vi "Intensity RMS.vi"(8 "Original Intensity":dbl[][](array[numeric]) format="%0.3f", 9 "Iteration":i32=9, 10 "num rows":i32=256, 11 "field":T1) -> (2 "Best Exponential Fit":dbl[](array[numeric]), 3 "field out":T1)   [LabVIEW 2012, in "LightPipes.lvlib"]
uses:
  LightPipes.lvlib
  <vilib>/Analysis/5stat.llb/RMS (DBL).vi
  <vilib>/Analysis/NI_AALPro.lvlib
  <vilib>/ptbypt/NI_PtbyPt.lvlib
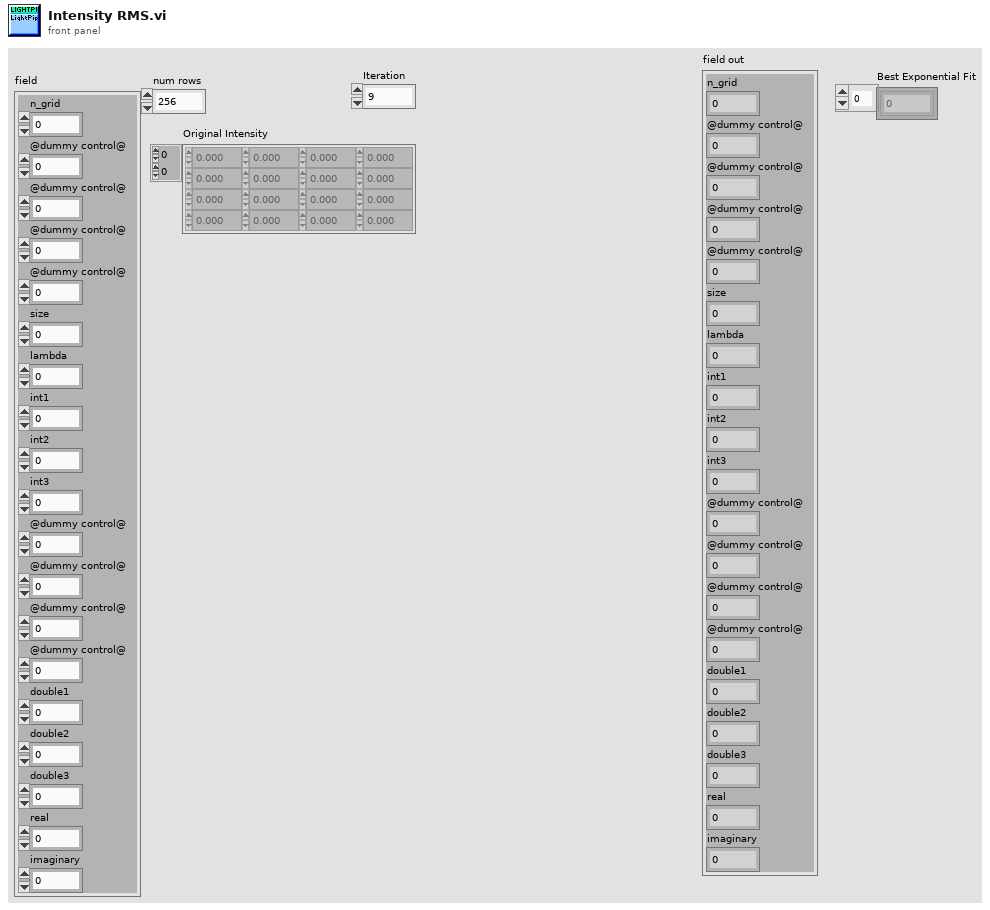
[diagram p1: front panel]
types:
  T1 = cluster{"n_grid":i32, "@dummy control@":i8, "@dummy control@":i8, "@dummy control@":i8, "@dummy control@":i8, "size":dbl, "lambda":dbl, "int1":i32, "int2":i32, "int3":i32, "@dummy control@":i8, "@dummy control@":i8, "@dummy control@":i8, "@dummy control@":i8, "double1":dbl, "double2":dbl, "double3":dbl, "real":u32, "imaginary":u32}
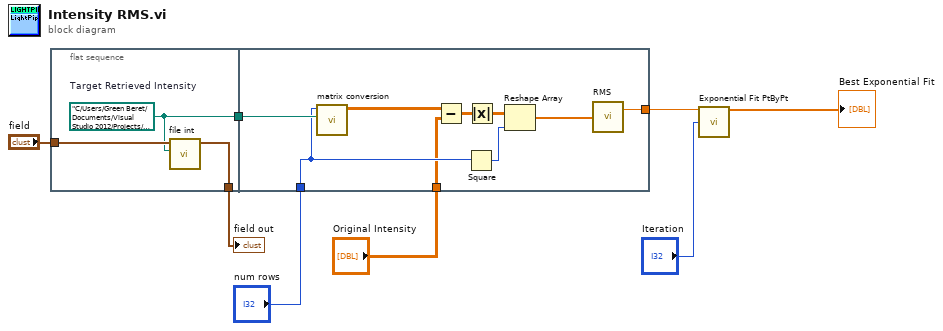
[diagram p0: block diagram]
diagram:
  n1 = flat-sequence {
    tunnel: "field" -> [w11]
    tunnel: [w9] -> w5
    tunnel: [w10] -> w8
    tunnel: "num rows" -> [w16]
    tunnel: w8 -> [w17]
    tunnel: "Original Intensity" -> [w13]
    tunnel: [w12] -> w2
    frame #0 {
      w10 = path "C:/Users/Green Beret/Documents/Visual Studio 2012/Projects/LightPipes/LightPipes/lp12src/LabView/images/target_retrieved_int.gpl"  # Target Retrieved Intensity
      n2 = call "file int.vi"("Path in"=w10, "field"=w11) -> ("field out"=w9:T1)  [unwired: 9 in]
    }
    frame #1 {
      n3 = call "matrix conversion.vi"("File Path"=w17, "number of rows (all:-1)"=w16) -> ("all rows"=w15:dbl[][])  [unwired: 9 in]
      n4 = Subtract(x=w15, y=w13) -> (x-y=w20:dbl[][])
      n5 = Square(x=w16) -> (x^2=w14:i32)
      n6 = Absolute Value(x=w20) -> (abs(x)=w19:dbl[][])
      n7 = Reshape Array "Reshape Array"(w19, w14) -> (w18:dbl[])
      n8 = call-poly <vilib>:"RMS.vi"("X"=w18) -> ("rms value"=w12:dbl)  [unwired: 1 out]
    }
  }
  n9 = call <vilib>:"Exponential Fit PtByPt.vi"("y"=w2, "x"="Iteration") -> ("Best Exponential Fit"=→"Best Exponential Fit":dbl[])  [unwired: 9 in, 4 out]
  "field out" <- w5
